vi "Regler Gaskuehler.vi"(8 "Fehler":errorcluster caption="Fehler (Eingang)") -> (0 "Fehler (Ausgang)":errorcluster)   [LabVIEW 2020, in "Regler.lvlib" / "Druckregler.lvlib"]
uses:
  Druckregler.lvlib
  Aktionen Param. Druckregler.ctl
  Konfig-Dateien/FGV Betriebsdaten Aktionen.ctl
  Verwaltung/FGV IN Aktionen.ctl
  Verwaltung/Verwaltung - cRIO.lvlib
  Konfig-Dateien/Konfig-Dateien.lvlib
  Allgemein/Allgemein.lvlib
  Verwaltung/FGV OUT Aktionen.ctl
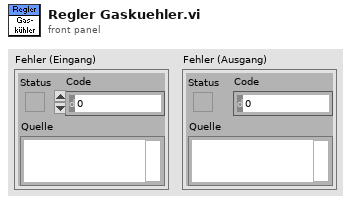
[diagram p1: front panel]
types:
  T1 = typedef "Regler.lvlib/Druckregler.lvlib/Aktionen Param. Druckregler.ctl" = enum16{"lesen", "schreiben", "Regler FT-IR", "Regler Ausgang", "Regler Durchfluss", "Regler PMA", "Regler NDIR", "Regler Filterblock", "Regler Gaskühler", "Regler Kalter Block"}
  T2 = typedef "Verwaltung - cRIO.lvlib/FGV IN Aktionen.ctl" = enum16{"lesen", "DI", "AI", "Fühler Br.", "TC", "Fühler Br. TC"}
  T3 = typedef "Konfig-Dateien.lvlib/FGV Betriebsdaten Aktionen.ctl" = enum16{"lesen", "Anlagengrenzw.", "PID Param.", "Sonstige", "Sensor Para."}
  T4 = typedef "Anlagengrenzwerte.lvlib/Anlagen-Grenzwerte Anzeige.ctl" = cluster{"Eingangsdruck FT-IR:":T5, "Durchfluss FT-IR:":T5, "Durchfluss CalGas:":T5, "Druck Ausgang:":T5, "Druck Kalter Block:":T5, "Heizleitungen intern:":T5, "Heizleitung zu FT-IR:":T5, "Heizung Filterblock:":T5, "Heizung Pumpe:":T5, "Heizleitung Extern SP1:":T5, "Heizleitung Extern SP2:":T5, "FT-IR Heizung Messzelle:":T5, "Schaltschranktemperatur:":T5, "Gaskühler:":T5}
  T5 = typedef "Anlagengrenzwerte.lvlib/Anlagen-Parameter Anzeige.ctl" = cluster{"Sollwert":sgl, "Warn-Min":sgl, "Warn-Max":sgl, "Abschalt-Min":sgl, "Abschalt-Max":sgl, "Regler":u16}
  T6 = typedef "Verwaltung - cRIO.lvlib/TC Eingaenge.ctl" = cluster{"TC0: Reserve":sgl, "TC1: HL zu FT-IR":sgl, "TC2: HL Extern SP1":sgl, "TC3: HL Extern SP2":sgl, "TC4: Reserve":sgl, "TC5: Reserve":sgl, "TC6: Reserve":sgl, "TC7: Reserve":sgl, "TC8: FT-IR":sgl, "TC9: Reserve":sgl, "TC10: Schaltschrank":sgl, "TC11: Umgebung":sgl}
  T7 = cluster{"Numerisch":sgl, "Numerisch":sgl, "Numerisch":sgl, "Numerisch":sgl, "Numerisch":sgl}
  T8 = typedef "Regler.lvlib/Druckregler.lvlib/Regler Interne Werte.ctl" = cluster{"PV":sgl, "D-action":sgl, "Error":sgl, "I-action":sgl, "OUT":sgl}
  T9 = typedef "Verwaltung - cRIO.lvlib/FGV OUT Aktionen.ctl" = enum16{"lesen", "ANA OUT", "DO 0-31", "DO 32-47"}
  T10 = typedef "Verwaltung - cRIO.lvlib/Digital Ausgaenge 32-63.ctl" = cluster{"O32: Messgaspumpe EIN":bool, "O33: (Umgebungsluftpumpe)":bool, "O34: (Kondensatpumpe GK)":bool, "O35: Klima/Lüfter EIN":bool, "O36: Versorgung Heizungen":bool, "O37: Versorgung Heizungen":bool, "O38: (Gaskühler EIN (Freigabe))":bool, "O39: Störung FAS LP":bool, "O40: (Heizung Filterblock)":bool, "O41: Heizung HL zu FT-IR":bool, "O42: Heizung HL Extern SP1":bool, "O43: Heizung HL Extern SP2":bool, "O44: Heizung Reserve":bool, "O45: Heizung Reserve":bool, "O46: Statusbeleuchtung grün":bool, "O47: Statusbeleuchtung rot":bool}
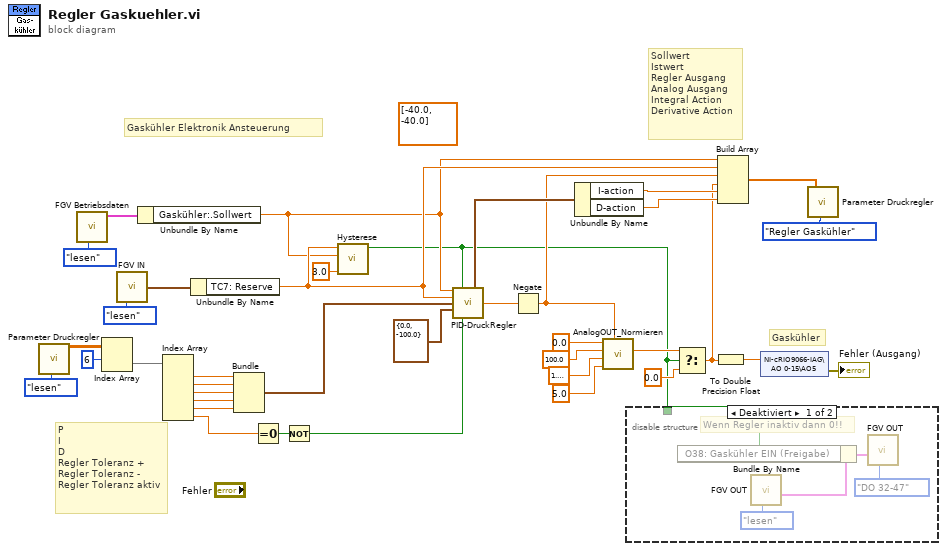
[diagram p0: block diagram]
diagram:
  (unwired) sgl[] [-40.0, -40.0] ("Regler Interne Werte")
  # "Gaskühler"
  # "Gaskühler Elektronik Ansteuerung"
  # "Sollwert\nIstwert\nRegler Ausgang\nAnalog Ausgang\nIntegral Action\nDerivative Action"
  # "P\nI\nD\nRegler Toleranz +\nRegler Toleranz -\nRegler Toleranz aktiv"
  n1 = call "Parameter Druckregler.vi"("Aktionen"=Aktionen_Param._Druckregler."lesen") -> ("Regleparameter"=w28:sgl[][])  [unwired: 10 in, 8 out]
  n2 = call "FGV Betriebsdaten.vi"("Aktionen"=FGV_Betriebsdaten_Aktionen."lesen") -> ("Anlagen-Grenzwerte"=w4:T4)  [unwired: 7 in, 3 out]
  n3 = Index Array(array=w28, index (row)=6 ("Deaktivierter Index (Spalte)")) -> (element=w29:sgl[])  [unwired: 1 in]
  n4 = call "FGV IN.vi"("Aktion"=FGV_IN_Aktionen."lesen") -> ("TC Eingänge"=w7:T6)  [unwired: 10 in, 4 out]
  n5 = Unbundle By Name(w4) -> ("Gaskühler:.Sollwert"=w12:sgl)
  n6 = Index Array(array=w29) -> (element #1=w19:sgl, element #2=w20:sgl, element #3=w21:sgl, element #4=w22:sgl, element #5=w23:sgl, element #6=w33:sgl)  [unwired: 6 in]
  n7 = Unbundle By Name(w7) -> ("TC7: Reserve"=w13:sgl)
  n8 = Bundle("Numerisch"=w19, "Numerisch"=w20, "Numerisch"=w21, "Numerisch"=w22, "Numerisch"=w23) -> (w25:T7)  [unwired: 1 in]
  n9 = Equal To 0?(x=w33) -> (x = 0?=w24:bool)
  n10 = Not(x=w24) -> (.not. x?=w26:bool)
  n11 = call "Hysterese.vi"("Abschaltung!?"=sgl 3.0, "soll"=w12, "ist"=w13) -> ("ein/aus"=w1:bool)  [unwired: 7 in, 1 out]
  n12 = call "PID-DruckRegler.vi"("Sollwert"=w12, "Regler EIN"=w1, "Istwert"=w13, "PID-Parameter"=w25, "output range"=cluster{"output high":sgl, "output low":sgl} {"output high"=0.0, "output low"=-100.0}, "Regler Toleranz verwenden?"=w26) -> ("Regler Interne Werte"=w14:T8, "Output"=w32:sgl)  [unwired: 7 in, 1 out]
  n13 = Negate(x=w32) -> (-x=w9:sgl)
  n14 = Unbundle By Name(w14) -> ("I-action"=w34:sgl, "D-action"=w35:sgl)
  n15 = call "AnalogOUT_Normieren.vi"("Analogwert"=w9, "Obergrenze"=sgl 5.0, "Untergrenze"=sgl 1.3, "Max Analogwert"=sgl 100.0, "Min Analogwert"=sgl 0.0) -> ("Normierter Wert"=w11:sgl)  [unwired: 6 in]
  n16 = disable-structure shown="Deaktiviert" {
    disable-tunnel: w1 -> [w39 _]
    frame Disabled {
      # "Wenn Regler inaktiv dann 0!!"
      n17 = call "FGV OUT.vi"("Aktion"=FGV_OUT_Aktionen."lesen") -> ("DO 32-63"=w41:T10)  [unwired: 7 in, 3 out]
      n18 = Bundle By Name(cluster=w41, "O38: Gaskühler EIN (Freigabe)"=w39) -> (w40:T10)
      n19 = call "FGV OUT.vi"("Aktion"=FGV_OUT_Aktionen."DO 32-47", "DO 32-63"=w40) -> ()  [unwired: 6 in, 4 out]
    }
    frame Enabled {
    }
  }
  n20 = Select(t=w11, s=w1, f=sgl 0.0) -> (s? t:f=w8:sgl)
  n21 = To Double Precision Float(number=w8) -> (double precision float=w31:dbl)
  n22 = Build Array(w12, w13, w9, w8, w34, w35) -> (w3:sgl[])
  n23 = shared-variable "NI-cRIO9066-IAG\\AO 0-15\\AO5"(w31) -> (error out=→"Fehler (Ausgang)":errorcluster)  [unwired: 1 in]
  n24 = call "Parameter Druckregler.vi"("Werte Gaskühler"=w3, "Aktionen"=Aktionen_Param._Druckregler."Regler Gaskühler") -> ()  [unwired: 9 in, 9 out]
